vi "Settrigger_input.vi"(8 "error in (no error)":errorcluster, 10 "Set_Val":T1, 11 "OneOfTemplate in":refnum<class "niswitch_grpc_ConfigureScanTriggerRequest_trigger_input_enum.lvclass">) -> (0 "error out":errorcluster, 3 "OneOfTemplate out":refnum<class "niswitch_grpc_ConfigureScanTriggerRequest_trigger_input_enum.lvclass">)   [LabVIEW 2021, in "NI Switch_client.lvlib" / "niswitch_grpc_ConfigureScanTriggerRequest_trigger_input_enum.lvclass"]
uses:
  niswitch_grpc_ConfigureScanTriggerRequest_trigger_input_enum.lvclass
  niswitch_grpc_TriggerInput.ctl
  niswitch_grpc_ConfigureScanTriggerRequest_trigger_input_enum.lvclass/niswitch_grpc_ConfigureScanTriggerRequest_trigger_input_enum.ctl
  NI Switch_client.lvlib
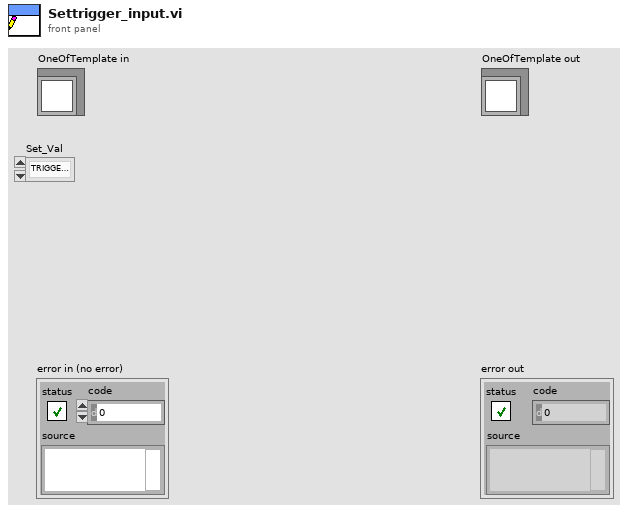
[diagram p1: front panel]
types:
  T1 = typedef "NI Switch_client.lvlib/niswitch_grpc_TriggerInput.ctl" = enum32{"TRIGGER_INPUT_UNSPECIFIED", "TRIGGER_INPUT_NISWITCH_VAL_IMMEDIATE", "TRIGGER_INPUT_NISWITCH_VAL_EXTERNAL", "TRIGGER_INPUT_NISWITCH_VAL_SOFTWARE_TRIG", "TRIGGER_INPUT_NISWITCH_VAL_TTL0", "TRIGGER_INPUT_NISWITCH_VAL_TTL1", "TRIGGER_INPUT_NISWITCH_VAL_TTL2", "TRIGGER_INPUT_NISWITCH_VAL_TTL3", "TRIGGER_INPUT_NISWITCH_VAL_TTL4", "TRIGGER_INPUT_NISWITCH_VAL_TTL5", "TRIGGER_INPUT_NISWITCH_VAL_TTL6", "TRIGGER_INPUT_NISWITCH_VAL_TTL7", "TRIGGER_INPUT_NISWITCH_VAL_PXI_STAR", "TRIGGER_INPUT_NISWITCH_VAL_REARCONNECTOR", "TRIGGER_INPUT_NISWITCH_VAL_FRONTCONNECTOR", "TRIGGER_INPUT_NISWITCH_VAL_REARCONNECTOR_MODULE1", "TRIGGER_INPUT_NISWITCH_VAL_REARCONNECTOR_MODULE2", "TRIGGER_INPUT_NISWITCH_VAL_REARCONNECTOR_MODULE3", "TRIGGER_INPUT_NISWITCH_VAL_REARCONNECTOR_MODULE4", "TRIGGER_INPUT_NISWITCH_VAL_REARCONNECTOR_MODULE5", "TRIGGER_INPUT_NISWITCH_VAL_REARCONNECTOR_MODULE6", "TRIGGER_INPUT_NISWITCH_VAL_REARCONNECTOR_MODULE7", "TRIGGER_INPUT_NISWITCH_VAL_REARCONNECTOR_MODULE8", "TRIGGER_INPUT_NISWITCH_VAL_REARCONNECTOR_MODULE9", "TRIGGER_INPUT_NISWITCH_VAL_REARCONNECTOR_MODULE10", "TRIGGER_INPUT_NISWITCH_VAL_REARCONNECTOR_MODULE11", "TRIGGER_INPUT_NISWITCH_VAL_REARCONNECTOR_MODULE12", "TRIGGER_INPUT_NISWITCH_VAL_FRONTCONNECTOR_MODULE1", "TRIGGER_INPUT_NISWITCH_VAL_FRONTCONNECTOR_MODULE2", "TRIGGER_INPUT_NISWITCH_VAL_FRONTCONNECTOR_MODULE3", "TRIGGER_INPUT_NISWITCH_VAL_FRONTCONNECTOR_MODULE4", "TRIGGER_INPUT_NISWITCH_VAL_FRONTCONNECTOR_MODULE5", "TRIGGER_INPUT_NISWITCH_VAL_FRONTCONNECTOR_MODULE6", "TRIGGER_INPUT_NISWITCH_VAL_FRONTCONNECTOR_MODULE7", "TRIGGER_INPUT_NISWITCH_VAL_FRONTCONNECTOR_MODULE8", "TRIGGER_INPUT_NISWITCH_VAL_FRONTCONNECTOR_MODULE9", "TRIGGER_INPUT_NISWITCH_VAL_FRONTCONNECTOR_MODULE10", "TRIGGER_INPUT_NISWITCH_VAL_FRONTCONNECTOR_MODULE11", "TRIGGER_INPUT_NISWITCH_VAL_FRONTCONNECTOR_MODULE12"}
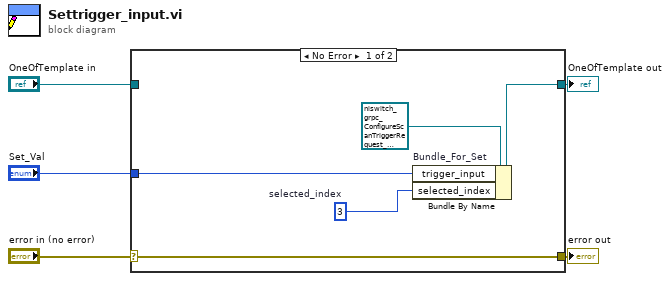
[diagram p0: block diagram]
diagram:
  n1 = case shown="No Error" "error in (no error)" {
    selector: "error in (no error)" -> [w10 w11]
    tunnel: [w10 w11] -> w4
    tunnel: [w9 w12] -> w2
    tunnel: "OneOfTemplate in" -> [_ w12]
    tunnel: "Set_Val" -> [w8 _]
    frame No Error {
      w7 = 3  # selected_index
      n2 = Bundle By Name "Bundle_For_Set"(cluster=refnum<class "niswitch_grpc_ConfigureScanTriggerRequest_trigger_input_enum.lvclass"> refnum ("OneOfTemplate in"), "trigger_input"=w8, "selected_index"=w7) -> (w9:refnum<class "niswitch_grpc_ConfigureScanTriggerRequest_trigger_input_enum.lvclass">)
    }
    frame Error {
    }
  }
  "error out" <- w4
  "OneOfTemplate out" <- w2
